vi "principal.vi"   [LabVIEW 2012, in "ExemploFinal.lvrbt"]
uses:
  ExemploFinal.lvrbt
  <vilib>/NXT/Subs/LVHSConnector.ctl
  <vilib>/NXT/LegoClasses/BrickReference/BrickReference.lvclass
  <vilib>/NXT/Remote Library/Sound/NXT_SoundVolume.ctl
  <vilib>/NXT/Dual Mode Library/Sound/PlaySoundFile.vi
  <vilib>/NXT/Dual Mode Library/Display/drawText_Center.vi
  <vilib>/NXT/Dual Mode Library/Waits/Wait_Num.vi
  <vilib>/NXT/Dual Mode Library/Sound/PlayC.vi
  <vilib>/NXT/Dual Mode Library/Sound/PlayB.vi
types:
  T1 = typedef "NXT_SoundVolume.ctl" = u8
  T2 = typedef "LVHSConnector.ctl" = refnum<class "BrickReference.lvclass">
  T3 = cluster{"TouchOUT":bool, "SomOUT":i32, "LuzOUT":i32, "UltrasomOUT":i32, "BotãoOUT":bool}
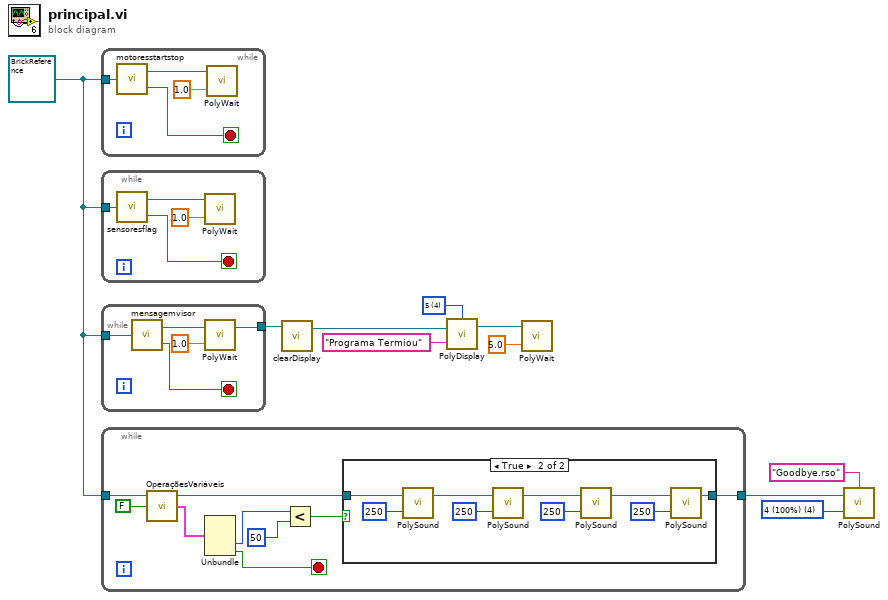
[diagram p0: block diagram]
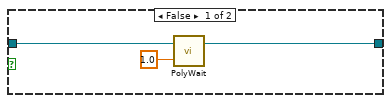
[diagram p2: hidden frame]
diagram:
  w8 = T1 4 items=["0 (Mute)", "1 (25%)", "2 (50%)", "3 (75%)", "4 (100%)"] ("Volume (4)")
  w10 = i16 4 items=["1", "2", "3", "4", "5", "6", "7", "8", "9", "10", "11", "12"] ("Line")
  w5 = T2 refnum ("NXT/EV3")
  n1 = while {
    tunnel: w5 -> [w13]
    stop <- w12 stop-if-true
    n2 = call "motoresstartstop.vi"("NXTIN"=w13) -> ("NXT OUT"=w11:T2, "FinalizarPrograma?"=w12:bool)
    n3 = call-poly <vilib>:"PolyWait.vi"("Time (1 sec)"=sgl 1.0, "NXT/EV3"=w11) -> ()  [unwired: 2 in, 1 out]
  }
  n4 = while {
    tunnel: w5 -> [w17]
    stop <- w15 stop-if-true
    n5 = call "sensoresflag.vi"("NXT IN"=w17) -> ("NXT OUT"=w16:T2, "FinalizarPrograma?"=w15:bool)
    n6 = call-poly <vilib>:"PolyWait.vi"("Time (1 sec)"=sgl 1.0, "NXT/EV3"=w16) -> ()  [unwired: 2 in, 1 out]
  }
  n7 = while {
    tunnel: w5 -> [w21]
    tunnel: [w22] -> w2
    stop <- w20 stop-if-true
    n8 = call "mensagemvisor.vi"("NXT IN"=w21) -> ("NXT OUT"=w19:T2, "FinalizarPrograma?"=w20:bool)
    n9 = call-poly <vilib>:"PolyWait.vi"("Time (1 sec)"=sgl 1.0, "NXT/EV3"=w19) -> ("NXT/EV3"=w22:T2)  [unwired: 2 in]
  }
  n10 = while {
    tunnel: w5 -> [w30]
    tunnel: [w27] -> w3
    stop <- w25 stop-if-true
    n11 = call "OperaçõesVariáveis.vi"("Escrever?"=FALSE, "NXT IN"=w30) -> ("Saídas"=w26:T3, "NXT OUT"=w29:T2)  [unwired: 1 in, 1 out]
    n12 = Unbundle(w26) -> ("UltrasomOUT"=w24:i32, "BotãoOUT"=w25:bool)  [unwired: 3 out]
    n13 = Less?(x=w24, y=50) -> (x < y?=w31:bool)
    n14 = case shown="True" w31 {
      tunnel: w29 -> [w35 w37]
      tunnel: [w34 w36] -> w27
      frame False {
        n15 = call-poly <vilib>:"PolyWait.vi"("Time (1 sec)"=sgl 1.0, "NXT/EV3"=w35) -> ("NXT/EV3"=w34:T2)  [unwired: 2 in]
      }
      frame True {
        n16 = call-poly <vilib>:"PolySound.vi"("Duration (500 ms)"=u16 250, "NXT/EV3"=w37) -> ("NXT/EV3"=w41:T2)  [unwired: 2 in]
        n17 = call-poly <vilib>:"PolySound.vi"("Duration (500 ms)"=u16 250, "NXT/EV3"=w41) -> ("NXT/EV3"=w38:T2)  [unwired: 2 in]
        n18 = call-poly <vilib>:"PolySound.vi"("Duration (500 ms)"=u16 250, "NXT/EV3"=w38) -> ("NXT/EV3"=w42:T2)  [unwired: 2 in]
        n19 = call-poly <vilib>:"PolySound.vi"("Duration (500 ms)"=u16 250, "NXT/EV3"=w42) -> ("NXT/EV3"=w36:T2)  [unwired: 2 in]
      }
    }
  }
  n20 = call <vilib>:"clearDisplay.vi"("NXT/EV3"=w2) -> ("NXT/EV3"=w1:T2)  [unwired: 3 in]
  n21 = call-poly <vilib>:"PolyDisplay.vi"("Text"="Programa Termiou", "NXT/EV3"=w1, "Line"=w10) -> ("NXT/EV3"=w4:T2)  [unwired: 1 in]
  n22 = call-poly <vilib>:"PolyWait.vi"("Time (1 sec)"=sgl 5.0, "NXT/EV3"=w4) -> ()  [unwired: 2 in, 1 out]
  n23 = call-poly <vilib>:"PolySound.vi"("Volume (4)"=w8, "NXT/EV3"=w3, "Filename (*.rso/*.rsf)"="Goodbye.rso") -> ()  [unwired: 1 in, 1 out]
